vi "ReadAnalog3_PulseWidth_FWHM.vi"() -> ()   [LabVIEW 2016]
doc: "Demonstrates the use of the Read/Write Control for communication between the FPGA target and host VI. This is the FPGA target VI. The controls and indicators on the front panel of this VI can be read by the host VI using the Read/Write Control function."
uses:
  <vilib>/rvi/Analysis/measure/period/templates/niFPGA Period Edge Direction.ctl
  <vilib>/Platform/TimedLoop/XDataNode/timing_clust.ctl
  <vilib>/Platform/TimedLoop/XDataNode/nitl_modes.ctl
  <vilib>/Platform/TimedLoop/XDataNode/wakeup.ctl
  <vilib>/rvi/Emulation/niFpgaGetClockAttributes.vi
  <vilib>/rvi/Emulation/niFpgaSctlEmulationGetInTimedLoop.vi
  <vilib>/rvi/Emulation/niFpgaEmulationReportErrorSimple.vi
  <vilib>/rvi/eio/common/nirviEmuTemplateMethod_errors.vi
  <vilib>/rvi/Analysis/common/codeGenErrors/XNode/niFpgaXNodeCodeGenErrorHandle.vi
  <vilib>/rvi/Emulation/niFpgaCriticalErrorInLSC.vi
  <vilib>/rvi/Analysis/utilities/niFPGA Threshold Crossing Logic.vi
  <vilib>/rvi/interface/RandomDataEmulation/niFpgaRandomDataHandleErrors.vi
  <vilib>/rvi/Emulation/niFpgaProcessEmulError.vi
  <vilib>/rvi/occurrence/nirviWaitOnOccurrenceBase.vi
  <vilib>/eio/EIONode/EIONode.xnode
  <vilib>/rvi/Analysis/measure/butterworth/XNode/niFpgaButterworthFilter.xnode
  <vilib>/rvi/Analysis/measure/period/XNode/niFpgaAnalogPeriod.xnode
  <vilib>/Platform/TimedLoop/XDataNode/XDataNode.xnode
  <vilib>/rvi/DataTransferAndStorage/Container/XNode/niFpgaContainer.xnode
  <vilib>/rvi/interface/RandomDataEmulation/nirviRandomDataFpgaReadWriteTemplate.vi
  <vilib>/Platform/TimedLoop/XDataNode/XDNodeRunTimeDep.lvlib
panel:
  in  "Trigger Length":u32 caption="Count(uSec)"
  in  "Sort":bool
  out "Event Count":u32
  in  "Count Reset":bool
  in  "Max Width":u32
  in  "Min Width":u32
  in  "Max Sorting Threshold":i16
  in  "Noise Level":i16
  in  "PMT Voltage":i16
  in  "Min Sorting Threshold":i16
  in  "Loop Period (ticks)":u32 caption="Count(Ticks)"
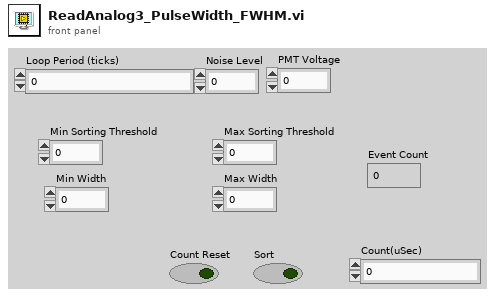
[diagram p1: front panel]
types:
  T1 = typedef "XDNodeRunTimeDep.lvlib/timing_clust.ctl" = cluster{"Expected End [f-1]":u64, "Actual End [f-1]":u64, "Finished Late? [f-1]":bool, "Expected End [i-1]":u64, "Actual End [i-1]":u64, "Finished Late? [i-1]":bool, "Expected Start [i]":u64, "Actual Start [i]":u64, "Expected Start [f]":u64, "Actual Start [f]":u64, "Source Name":string, "Structure Name":string, "Period":i64, "Deadline":i64, "Offset":i64, "Start":i64, "Priority":i32, "Timeout":i32, "Mode":T2, "Wakeup Reason":T3, "Error":errorcluster, "Source Type":string, "Secondary Source Type":string, "Global End Time":u64, "Global Start Time":u64, "Frame Duration":u64, "Iteration Duration":u64, "Assigned CPU":i32, "I/O Scan Engine Mode":u32}
  T2 = typedef "XDNodeRunTimeDep.lvlib/nitl_modes.ctl" = enum32{"No Change", "Process missed periods, maintain original phase", "Discard missed periods, maintain original phase", "Process missed periods, ignore original phase", "Discard missed periods, ignore original phase"}
  T3 = typedef "XDNodeRunTimeDep.lvlib/wakeup.ctl" = enum32{"Normal", "Aborted", "Asynchronous wakeup", "Timing source error", "Timed loop error", "Timeout"}
  T4 = typedef "niFPGA Period Edge Direction.ctl" = u8
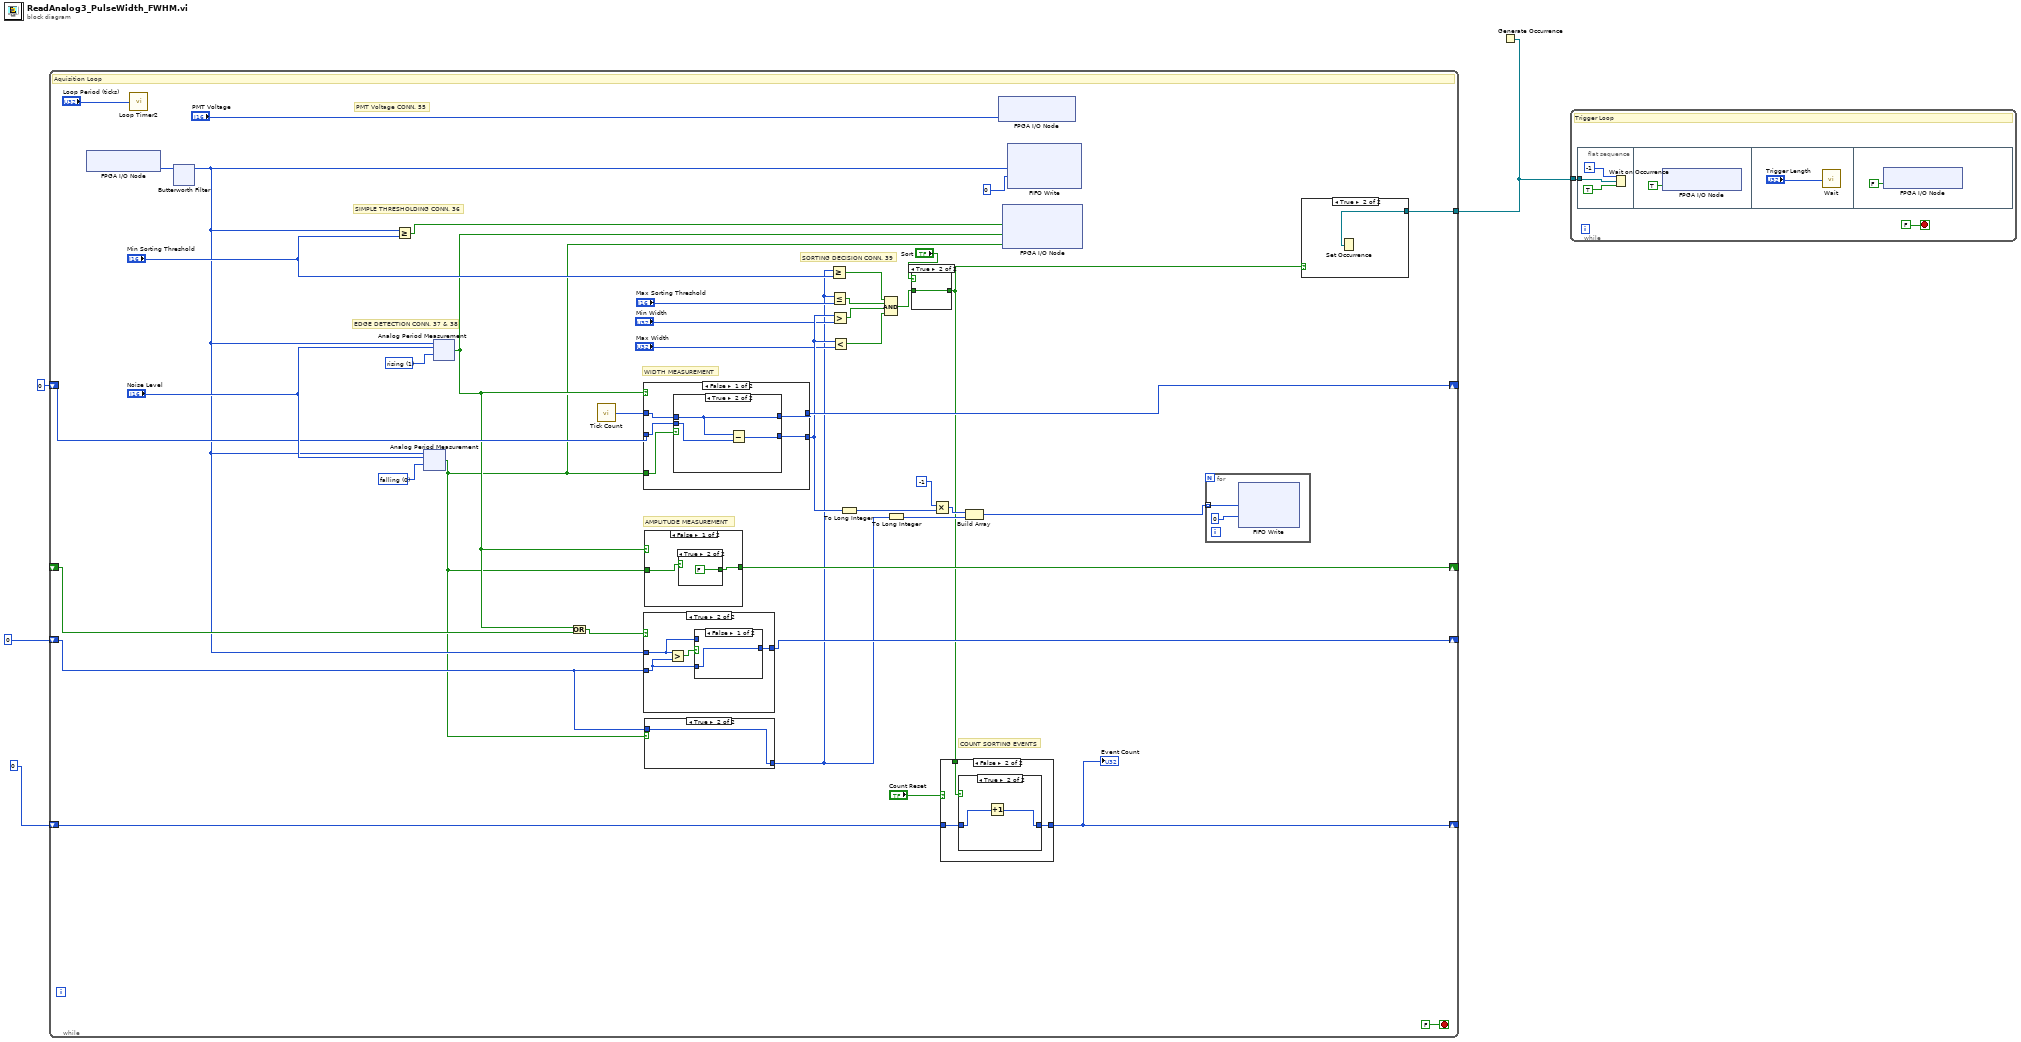
[diagram p0: block diagram]
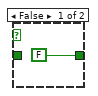
[diagram p3: hidden frame]
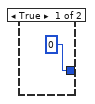
[diagram p4: hidden frame]
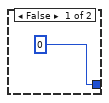
[diagram p6: hidden frame]
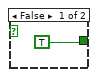
[diagram p7: hidden frame]
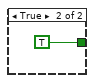
[diagram p8: hidden frame]
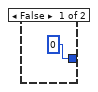
[diagram p9: hidden frame]
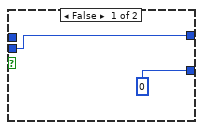
[diagram p11: hidden frame]
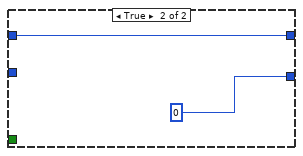
[diagram p12: hidden frame]
diagram:
  n1 = Generate Occurrence() -> (w1:refnum<k4>)
  n2 = while {
    shift-right: [w38] -> _
    shift-left: u32 0 ("Tick Count(uSec)") -> [w37]
    shift-right: [w34] -> _
    shift-left: i16 0 -> [w33]
    shift-right: [w36] -> _
    shift-left: _ -> [w35]
    shift-right: [w21] -> _
    shift-left: u32 0 -> [w22]
    tunnel: w1 -> [w5]
    stop <- FALSE stop-if-true
    w41 = T4 0 items=["falling", "rising"] ("direction")
    w42 = T4 1 items=["falling", "rising"] ("direction")
    # "COUNT SORTING EVENTS"
    # "PMT Voltage CONN. 55"
    # "SIMPLE THRESHOLDING CONN. 36"
    # "EDGE DETECTION CONN. 37 & 38"
    # "SORTING DECISION CONN. 39"
    # "AMPLITUDE MEASUREMENT"
    # "WIDTH MEASUREMENT"
    # "Aquisition Loop"
    n3 = xnode "FPGA I/O Node"() -> ("Connector0/AI0"=w10:i16)  [unwired: 1 in, 1 out]
    n4 = call "Loop Timer2"("Count(Ticks)"="Loop Period (ticks)") -> ()  [unwired: 1 out]
    n5 = xnode "Butterworth Filter"("input data"=w10) -> ("output data"=w9:i16)  [unwired: 2 in]
    n6 = Greater Or Equal?(x=w9, y="Min Sorting Threshold") -> (x >= y?=w45:bool)
    n7 = xnode "Analog Period Measurement"("input data"=w9, "threshold level"="Noise Level", "direction"=w41) -> ("crossing"=w7:bool)  [unwired: 2 in, 3 out]
    n8 = xnode "Analog Period Measurement"("input data"=w9, "threshold level"="Noise Level", "direction"=w42) -> ("crossing"=w17:bool)  [unwired: 2 in, 3 out]
    n9 = Or(x=w17, y=w35) -> (x .or. y?=w18:bool)
    n10 = call "Tick Count"() -> ("Tick Count(uSec)"=w39:u32)
    n11 = case shown="False" w17 {
      tunnel: w39 -> [w84 w92]
      tunnel: [w82 w92] -> w38
      tunnel: w37 -> [w83 _]
      tunnel: w7 -> [w85 _]
      tunnel: [w81 u32 0] -> w28
      frame False {
        n12 = case shown="True" w85 {
          tunnel: w84 -> [_ w89]
          tunnel: w83 -> [w87 w90]
          tunnel: [w87 w89] -> w82
          tunnel: [u32 0 w88] -> w81
          frame False {
          }
          frame True {
            n13 = Subtract(x=w89, y=w90) -> (x-y=w88:u32)
          }
        }
      }
      frame True {
      }
    }
    n14 = case shown="True" w18 {
      tunnel: w9 -> [_ w77]
      tunnel: w33 -> [_ w75]
      tunnel: [i16 0 ("Connector0/AI0") w76] -> w34
      frame False {
      }
      frame True {
        n15 = Greater?(x=w77, y=w75) -> (0:w78:bool)
        n16 = case shown="False" w78 {
          tunnel: w77 -> [_ w80]
          tunnel: [w79 w80] -> w76
          tunnel: w75 -> [w79 _]
          frame False {
          }
          frame True {
          }
        }
      }
    }
    n17 = case shown="False" w17 {
      tunnel: [w69 TRUE ("crossing")] -> w36
      tunnel: w7 -> [w70 _]
      frame False {
        n18 = case shown="True" w70 {
          tunnel: [TRUE FALSE] -> w69
          frame False {
          }
          frame True {
          }
        }
      }
      frame True {
      }
    }
    n19 = case shown="True" w7 {
      tunnel: w33 -> [_ w68]
      tunnel: [i16 0 ("Connector0/AI0") w68] -> w8
      frame False {
      }
      frame True {
      }
    }
    n20 = Greater Or Equal?(x=w8, y="Min Sorting Threshold") -> (x >= y?=w32:bool)
    n21 = Less Or Equal?(x=w8, y="Max Sorting Threshold") -> (x <= y?=w31:bool)
    n22 = Greater?(x=w28, y="Min Width") -> (0:w30:bool)
    n23 = Less?(x=w28, y="Max Width") -> (x < y?=w29:bool)
    n24 = To Long Integer(number=w28) -> (32bit integer=w14:i32)
    n25 = Compound Arithmetic op=AND(w32, w31, w30, w29) -> (w20:bool)
    n26 = To Long Integer(number=w8) -> (32bit integer=w15:i32)
    n27 = case shown="True" "Sort" {
      tunnel: w20 -> [_ w59]
      tunnel: [FALSE w59] -> w11
      frame False {
      }
      frame True {
      }
    }
    n28 = Multiply(x=-1, y=w14) -> (x*y=w13:i32)
    n29 = case shown="False" "Count Reset" {
      tunnel: w11 -> [_ w63]
      tunnel: w22 -> [_ w62]
      tunnel: [u32 0 w61] -> w21
      frame True {
      }
      frame False {
        n30 = case shown="True" w63 {
          tunnel: w62 -> [w64 w66]
          tunnel: [w64 w65] -> w61
          frame False {
          }
          frame True {
            n31 = Increment(x=w66) -> (x+1=w65:u32)
          }
        }
      }
    }
    "Event Count" <- w21
    n32 = Build Array(w13, w15) -> (w6:i32[])
    n33 = xnode "FPGA I/O Node"("Connector0/AO0"="PMT Voltage") -> ()  [unwired: 2 in, 2 out]
    n34 = xnode "FPGA I/O Node"("Connector0/DIO0"=w45, "Connector0/DIO1"=w17, "Connector0/DIO2"=w7) -> ()  [unwired: 4 in, 4 out]
    n35 = xnode ("FIFO Write")("Element"=w9, "Timeout"=0) -> ()  [unwired: 1 in, 2 out]
    n36 = for {
      tunnel: w6 -> [w48] mode=indexing
      n37 = xnode ("FIFO Write")("Element"=w48, "Timeout"=0) -> ()  [unwired: 1 in, 2 out]
    }
    n38 = case shown="True" w11 {
      tunnel: w5 -> [_ w57]
      frame False {
      }
      frame True {
        n39 = Set Occurrence(w57) -> ()
      }
    }
  }
  n40 = while "Trigger Loop" {
    tunnel: w1 -> [w328]
    stop <- FALSE stop-if-true
    # "Trigger Loop"
    n41 = flat-sequence {
      tunnel: w328 -> [w331]
      frame #0 {
        n42 = Wait on Occurrence(1:TRUE ("ignore previous (T)"), 2:w331, 3:-1 ("ms timeout (-1)")) -> ()  [unwired: 1 out]
      }
      frame #1 {
        n43 = xnode "FPGA I/O Node"("Connector0/DIO3"=TRUE) -> ()  [unwired: 1 in, 1 out]
      }
      frame #2 {
        n44 = call "Wait"("Count(uSec)"="Trigger Length") -> ()  [unwired: 1 out]
      }
      frame #3 {
        n45 = xnode "FPGA I/O Node"("Connector0/DIO3"=FALSE) -> ()  [unwired: 1 in, 1 out]
      }
    }
  }
